vi "mono_simulator.vi"() -> ()   [LabVIEW 2018]
uses:
  mono_config_lidar.ctl
panel:
  out "camera_out":picture
  out "camera response":string
  in  "stop":bool
  out "error out":errorcluster
  out "vehicle drive response":string
  in  "right_amount":dbl(knob) scale=-1.0..1.0
  in  "forward_amount":dbl(slide) scale=-1.0..1.0
  out "vehicle command response":string
  in  "monoDrive Control Port":i32=8998
  in  "monoDrive Simulator IP":string="127.0.0.1"
  in  "Vehicle Configuration Path":path=path "C:/Users/celit/Documents/GitHub/client/configurations/vehicle/demo_vehicle"
  out "simulator config response":string
  in  "Simulator Configuration Path":path=path "C:/Users/celit/Documents/GitHub/client/configurations/simulator.json"
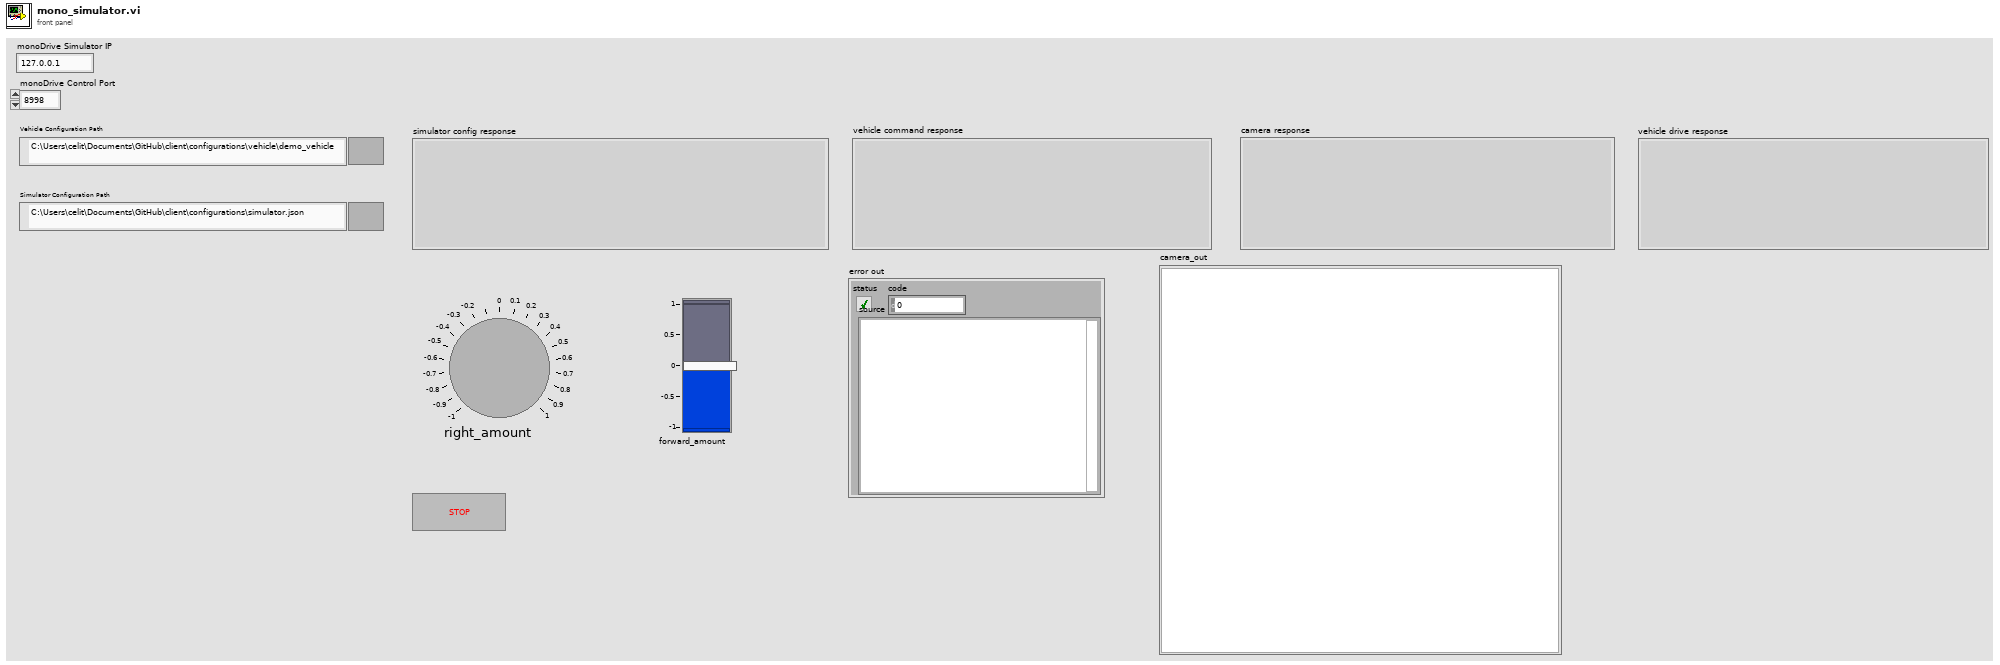
[diagram p1: front panel]
types:
  T1 = typedef "mono_config_lidar.ctl" = cluster{"type":string, "id":string, "packet_size":i32, "listen_port":i32, "display_process":bool, "sensor_process":bool, "synchronized_display":bool, "location":cluster{string, string, "z":i32}, "rotation":cluster{"pitch":i32, "yaw":i32, "roll":i32}, "max_distance":i32, "vertical_fov_angle":i32, "horizontal_resolution":i32, "fps":i32, "n_lasers":i32, "reset_angle":i32}
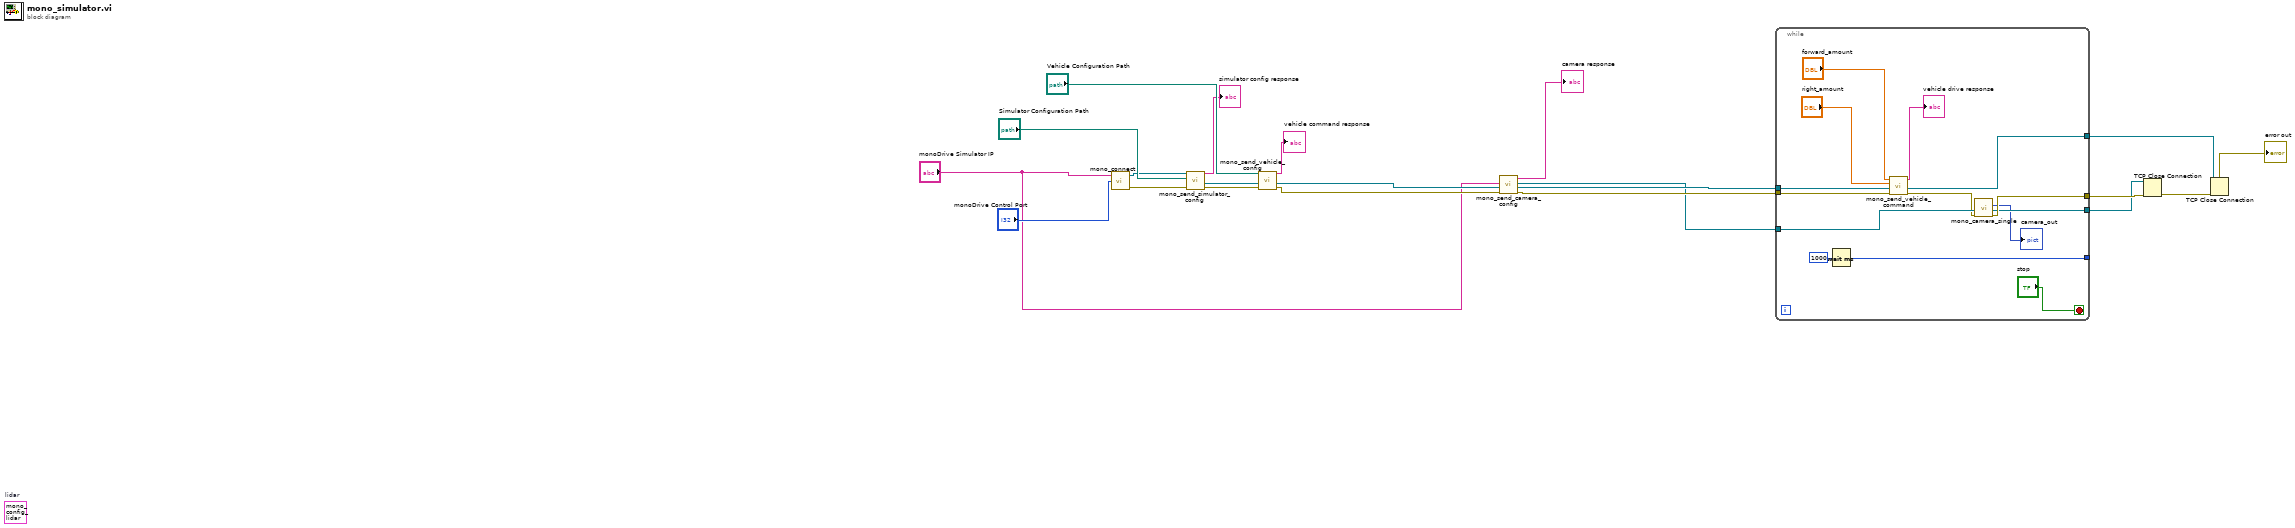
[diagram p0: block diagram]
diagram:
  (unwired) T1 {"type"="", "id"="", "packet_size"=0, "listen_port"=0, "display_process"=FALSE, "sensor_process"=FALSE, "synchronized_display"=FALSE, "location"={"", "", "z"=0}, "rotation"={"pitch"=0, "yaw"=0, "roll"=0}, "max_distance"=0, "vertical_fov_angle"=0, "horizontal_resolution"=0, "fps"=0, "n_lasers"=0, "reset_angle"=0}  # lidar
  n1 = call "mono_connect.vi"("monoDrive Control Port"="monoDrive Control Port", "monoDrive Simulator IP"="monoDrive Simulator IP") -> ("error out"=w16:errorcluster, "monoDrive Connection"=w17:refnum<k5>)  [unwired: 2 in]
  n2 = call "mono_send_simulator_config.vi"("error in"=w16, "Simulator Configuration Path"="Simulator Configuration Path", "monoDrive Connection In"=w17) -> ("error out"=w14:errorcluster, "monoDrive Connection Out"=w13:refnum<k5>, "data out"=→"simulator config response":string)  [unwired: 2 in]
  n3 = call "mono_send_vehicle_config.vi"("error in (no error)"=w14, "monoDrive Connection In"=w13, "Vehicle Configuration Path"="Vehicle Configuration Path") -> ("error out"=w10:errorcluster, "monoDrive Connection Out"=w9:refnum<k5>, "vehicle command response"=→"vehicle command response":string)  [unwired: 2 in]
  n4 = call "mono_send_camera_config.vi"("error in"=w10, "TCP Network Connection in"=w9, "simulator ip"="monoDrive Simulator IP") -> ("error out"=w7:errorcluster, "TCP Network Connection out"=w6:refnum<k5>, "sensor connection ID"=w4:refnum<k5>, "config response"=→"camera response":string)  [unwired: 1 in]
  n5 = while {
    tunnel: [w27] -> _
    tunnel: w7 -> [w30]
    tunnel: [w24] -> w3
    tunnel: w6 -> [w29]
    tunnel: [w35] -> w12
    tunnel: w4 -> [w26]
    tunnel: [w23] -> w1
    stop <- "stop" stop-if-true
    n6 = Wait (ms)(milliseconds to wait=u32 1000) -> (millisecond timer value=w27:u32)
    n7 = call "mono_send_vehicle_command.vi"("error in (no error)"=w30, "TCP Network Connection in"=w29, "right_amount"="right_amount", "forward_amount"="forward_amount") -> ("error out"=w25:errorcluster, "TCP Network Connection out"=w35:refnum<k5>, "vehicle command response 2"=→"vehicle drive response":string)  [unwired: 1 in]
    n8 = call "mono_camera_single.vi"("error in"=w25, "connection ID"=w26) -> ("error out"=w24:errorcluster, "tcp_out"=w23:refnum<k5>, "camera_out"=→"camera_out":picture)  [unwired: 3 in]
  }
  n9 = TCP Close Connection(connection ID=w1, error in (no error)=w3) -> (error out=w2:errorcluster)  [unwired: 1 in, 1 out]
  n10 = TCP Close Connection(connection ID=w12, error in (no error)=w2) -> (error out=→"error out":errorcluster)  [unwired: 1 in, 1 out]
